vi "ROS_Topic_Close_Primitive.vi"(2 "error in":errorcluster, 3 "ROS in":T1) -> (0 "error out":errorcluster)   [LabVIEW 2010]
uses:
  <userlib>/ROSforLV_0.1/ROS/Code/SubVIs/_ROSControl.ctl
  <userlib>/ROSforLV_0.1/ROS/Code/SubVIs/_ROSDirection.ctl
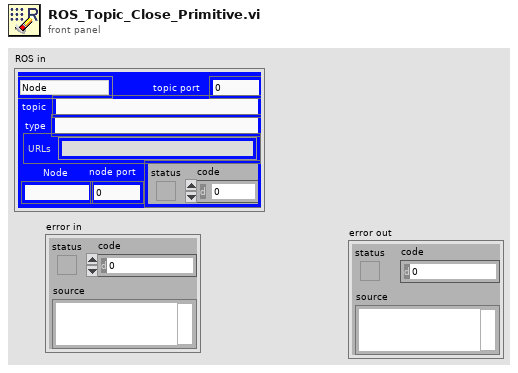
[diagram p1: front panel]
types:
  T1 = typedef "_ROSControl.ctl" = cluster{"topic port":u16, "Node":string, "topic":string, "type":string, "node port":u32, "error ":errorcluster, "Direction":T2, "APIs":string[]}
  T2 = typedef "_ROSDirection.ctl" = enum16{"Node", "Publisher", "Subscriber", "Service Client"}
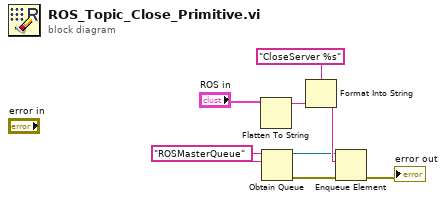
[diagram p0: block diagram]
diagram:
  w7 = "ROSMasterQueue" ("name (unnamed)")
  n1 = Flatten To String(anything="ROS in") -> (data string=w3:string)  [unwired: 3 in, 2 out]
  n2 = Obtain Queue(name (unnamed)=w7, element data type=w7) -> (queue out=w4:refnum<queue>, error out=w2:errorcluster)  [unwired: 3 in, 1 out]
  n3 = Format Into String(format string="CloseServer %s", w3) -> (resulting string=w5:string)  [unwired: 2 in, 1 out]
  n4 = Enqueue Element(queue=w4, element=w5, error in (no error)=w2) -> (error out=→"error out":errorcluster)  [unwired: 1 in, 2 out]
